vi "Read Interlock Status.vi"(8 "error in (no error)":errorcluster, 11 "Door Hardware in":refnum<class "Door Hardware.lvclass">) -> (0 "error out":errorcluster, 3 "Door Hardware out":refnum<class "Door Hardware.lvclass">)   [LabVIEW 2020, in "Door Hardware.lvlib" / "Door Hardware.lvclass"]
uses:
  Door Hardware.lvclass
  C:/Program Files/National Instruments/LabVIEW 2020/vi.lib/ActorFramework/Actor/Actor.lvclass
  Door Hardware.lvclass/Door Hardware.ctl
  <vilib>/ActorFramework/Actor/Actor.lvclass/Actor.ctl
  Door Controller API/Door Controller API Messages/Mode of Operation Value Change Msg/Mode of Operation Value Change Msg.lvclass/Mode of Operation Value Change Msg.ctl
  <vilib>/ActorFramework/Message Enqueuer/Message Enqueuer.lvclass/Message Enqueuer.ctl
  Door Controller API/Door Controller API Messages/Door Closed Interlock Value Change Msg/Door Closed Interlock Value Change Msg.lvclass/Door Closed Interlock Value Change Msg.ctl
  Door Controller API/Door Controller API Messages/Door Open Interlock Value Change Msg/Door Open Interlock Value Change Msg.lvclass/Door Open Interlock Value Change Msg.ctl
  <vilib>/ActorFramework/Message Enqueuer/Enqueue.vi
  Door Controller API/Door Controller API Messages/Mode of Operation Value Change Msg/Mode of Operation Value Change Msg.lvclass
  C:/Program Files/National Instruments/LabVIEW 2020/vi.lib/ActorFramework/Message/Message.lvclass
  Door Controller API/Door Controller API Messages/Door Closed Interlock Value Change Msg/Door Closed Interlock Value Change Msg.lvclass
  Door Controller API/Door Controller API Messages/Door Open Interlock Value Change Msg/Door Open Interlock Value Change Msg.lvclass
  <vilib>/ActorFramework/Message Priority Queue/Priority Enqueue.vi
  Door Interlocks/Door Interlocks.lvclass
  <vilib>/ActorFramework/Actor/Actor.lvclass
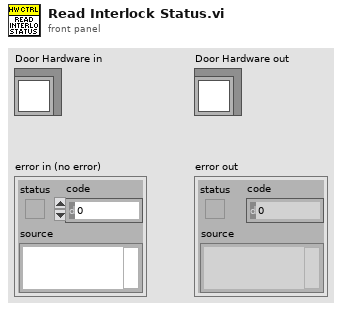
[diagram p1: front panel]
types:
  T1 = typedef "Door Interlocks.lvclass/Interlock Values.ctl" = cluster{"Door Open":bool, "Door Closed":bool, "Mode of Operation":T2}
  T2 = typedef "Door Interlocks.lvclass/Mode of Operation.ctl" = enum16{"Standard", "Interlock Override"}
  T3 = cluster{"Door Open":bool, "Door Closed":bool, "Mode of Operation":bool}
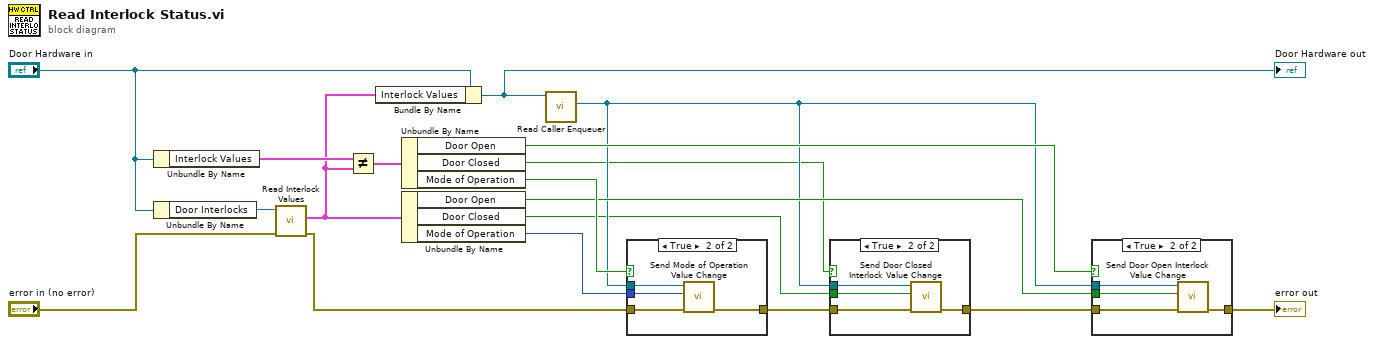
[diagram p0: block diagram]
diagram:
  n1 = Unbundle By Name("Door Hardware in") -> ("Interlock Values"=w16:T1)
  n2 = Unbundle By Name("Door Hardware in") -> ("Door Interlocks"=w18:refnum<class "Door Interlocks.lvclass">)
  n3 = call-dynamic "Read Interlock Values.vi"("error in (no error)"="error in (no error)", "Door Interlocks in"=w18) -> ("error out"=w4:errorcluster, "Interlock Values"=w3:T1)  [unwired: 8 in]
  n4 = Not Equal?(x=w16, y=w3) -> (x != y?=w15:T3)
  n5 = Bundle By Name(cluster="Door Hardware in", "Interlock Values"=w3) -> (w1:refnum<class "Door Hardware.lvclass">)
  "Door Hardware out" <- w1
  n6 = Unbundle By Name(w15) -> ("Door Open"=w12:bool, "Door Closed"=w9:bool, "Mode of Operation"=w14:bool)
  n7 = Unbundle By Name(w3) -> ("Door Open"=w11:bool, "Door Closed"=w8:bool, "Mode of Operation"=w13:T2)
  n8 = call <vilib>:"Read Caller Enqueuer.vi"("Actor"=w1) -> ("Caller Enqueuer"=w10:refnum<class "Message Enqueuer.lvclass">)  [unwired: 10 in]
  n9 = case shown="True" w14 {
    tunnel: w13 -> [_ w23]
    tunnel: w10 -> [_ w22]
    tunnel: [w19 w21] -> w7
    tunnel: w4 -> [w19 w20]
    frame False {
    }
    frame True {
      n10 = call "Send Mode of Operation Value Change.vi"("error in (no error)"=w20, "Mode of Operation"=w23, "Message Enqueuer"=w22) -> ("error out"=w21:errorcluster)  [unwired: 7 in, 1 out]
    }
  }
  n11 = case shown="True" w9 {
    tunnel: w10 -> [_ w28]
    tunnel: w7 -> [w24 w26]
    tunnel: w8 -> [_ w25]
    tunnel: [w24 w27] -> w6
    frame False {
    }
    frame True {
      n12 = call "Send Door Closed Interlock Value Change.vi"("error in (no error)"=w26, "Door Closed Interlock"=w25, "Message Enqueuer"=w28) -> ("error out"=w27:errorcluster)  [unwired: 7 in, 1 out]
    }
  }
  n13 = case shown="True" w12 {
    tunnel: w10 -> [_ w33]
    tunnel: w6 -> [w29 w32]
    tunnel: w11 -> [_ w31]
    tunnel: [w29 w30] -> w5
    frame False {
    }
    frame True {
      n14 = call "Send Door Open Interlock Value Change.vi"("error in (no error)"=w32, "Door Open Interlock"=w31, "Message Enqueuer"=w33) -> ("error out"=w30:errorcluster)  [unwired: 7 in, 1 out]
    }
  }
  "error out" <- w5
